vi "EnFlo_Hub.vi"() -> ()   [LabVIEW 2012]
uses:
  Anemometry Sub Vis/Controls/Launch_controls/Open_Calib.ctl
  Anemometry Sub Vis/Controls/Launch_controls/Open_Meas.ctl
  Anemometry Sub Vis/Controls/Launch_controls/Open_Enter_Temp.ctl
  Anemometry Sub Vis/Controls/Launch_controls/Multi_Run_Prog.ctl
  Anemometry Sub Vis/Controls/Launch_controls/EnFlo_arm.ctl
  Anemometry Sub Vis/Controls/Launch_controls/Fast_FID_Valve.ctl
  Anemometry Sub Vis/Controls/Launch_controls/Disp_Setup.ctl
  Anemometry Sub Vis/Controls/Launch_controls/EnFlo_Tun_Setup.ctl
  Anemometry Sub Vis/Controls/Launch_controls/User_Metadata.ctl
  Anemometry Sub Vis/Controls/Launch_controls/Trav_3D_move.ctl
  Anemometry Sub Vis/Controls/Launch_controls/Trav_Space.ctl
  Anemometry Sub Vis/Controls/Launch_controls/Tunnel_speed.ctl
  Anemometry Sub Vis/Controls/Launch_controls/Client_source_control.ctl
  Anemometry Sub Vis/Controls/Launch_controls/Hydrosonic_Manual.ctl
  Anemometry Sub Vis/Controls/Launch_controls/Preference_Panel.ctl
  Anemometry Sub Vis/Controls/Launch_controls/Hot_wire_Calculator.ctl
  Anemometry Sub Vis/Controls/Launch_controls/RW_X_Parker_Config.ctl
  Anemometry Sub Vis/Controls/Launch_controls/LDA_Alignment.ctl
  Anemometry Sub Vis/Controls/Launch_controls/Named_Serial_Comms.ctl
  Anemometry Sub Vis/Controls/Launch_controls/BSA_data_rates.ctl
  Anemometry Sub Vis/Controls/Launch_controls/Serial_Setup.ctl
  Anemometry Sub Vis/Controls/Launch_controls/Post_Process_icon.ctl
  Anemometry Sub Vis/Controls/Launch_controls/Edit_Ascii_file.ctl
  Anemometry Sub Vis/Controls/Launch_controls/Edit_Raw_DF.ctl
  Anemometry Sub Vis/Controls/Launch_controls/Results_file_plotter.ctl
  Anemometry Sub Vis/Controls/Launch_controls/Serial_Port_Names.ctl
  Anemometry Sub Vis/Controls/Launch_controls/Paul.ctl
  Anemometry Sub Vis/Controls/Launch_controls/Tom.ctl
  Anemometry Sub Vis/Controls/Launch_controls/Scani_Valve.ctl
  Anemometry Sub Vis/Controls/Launch_controls/Edit_sever_Channel.ctl
  Anemometry Sub Vis/Controls/Launch_controls/Day_file_plotter.ctl
  Anemometry Sub Vis/Controls/Launch_controls/Plot_Sever_Data.ctl
  Anemometry Sub Vis/Controls/Launch_controls/Adam_Table.ctl
  Anemometry Sub Vis/Controls/Launch_controls/Active_Channel_Control.ctl
  Anemometry Sub Vis/Controls/Setup.ctl
  Anemometry Sub Vis/Controls/Post_Process.ctl
  Anemometry Sub Vis/Controls/Preference_Mode.ctl
  Anemometry Sub Vis/Gen Trav/Trav_mode.ctl
  Anemometry Sub Vis/Controls/User_Specific_mode.ctl
  Anemometry Sub Vis/File/Setup_Filetype.ctl
  Anemometry Sub Vis/Calibration/Calib_mode.ctl
  Anemometry Sub Vis/Controls/Server_Comms.ctl
  Anemometry Sub Vis/Controls/App_Global.ctl
  Anemometry Sub Vis/Globals/Dynamic_call_global.ph.vi
  Anemometry Sub Vis/Globals/Constants_global.vi
  Anemometry Sub Vis/Globals/Preference_global.vi
  Anemometry Sub Vis/Globals/Meas_global.vi
  <vilib>/Platform/browser.llb/Open URL in Default Browser (string).vi
  Anemometry Sub Vis/Globals/Trav_pos_global.vi
  Anemometry Sub Vis/Acquisition/PWA/PWAtasksGLOBAL.vi
  Anemometry Sub Vis/Utilities/Email_transfer_global.vi
panel:
  out "List of ADAM channels to view":string[](array[string])
  out "List of ADAM control channels":string[](array[string])
  out "Analogue Dev Name":string="Dev2"
  out "Numeric":i32
  out "Rig Name":string="EnFlo Tunnel"
  out "All Users":path=path "/System Folder/Preferences/LabVIEW (EnFlo specific)/Meas Setups"
  out "Dummy Measurement":bool
  in  "stop":bool
  in  "Tab Control":T1(tab)
  in  "Tunnel Speed Control":T2
  in  "Traverse Space":T3
  in  "Trav 3D Move":T4 caption="3D Traverse Move"
  in  "User Metadata":T5
  in  "Multi Run Prog":T6
  in  "Enter Temp_Press":T7
  in  "Measurement Prog":T8 caption="Measurement"
  in  "Calibration Prog":T9 caption="Calibration"
  in  "Scani Valve":T10
  in  "LDA Alignment":T11
  in  "Hydrosonic Control":T12
  in  "Fast FID Valve":T13
  in  "Source Control":T14
  in  "Gas Release Setup":T15
  in  "EnFlo Tunnel Setup":T16
  in  "Heater Setup":bool caption="Inlet heater File"
  in  "EnFlo Arm":T17
  in  "EnFlo Tun Display":bool
  in  "Rig_Control":cluster{"Ch Name":string, "Boolean":bool}[](array[cluster])
  in  "ADAM Channels Control":T18 caption="Change Active Channels"
  in  "ADAM Scan Table":T19 caption="Run ADAM Scan Table"
  in  "Edit Server Channel":T20
  in  "Plot Server Channels":T21 caption="Plot Server Data"
  in  "Day Files Plotter":T22 caption="Plot Data From File"
  out "Current Values":cluster{"Ch Name":string, "Numeric":dbl}[](array[cluster])
  in  "Results File Plotter":T23
  in  "Edit Raw Data Files":T24
  in  "Edit ASCII File":T25
  in  "Post Process Raw Data":T26
  in  "Top Level Traverse":bool
  in  "Show Manual Sync":bool
  in  "Sync to server now":bool
  in  "Port Names":T27
  in  "Serial Setup":T28
  in  "LDA Data Rate":T29
  in  "Named Serial Comms":T30
  in  "RW Trav Setup":T31
  in  "Hot Wire Calc":T32
  in  "Preference Panel":T33
  in  "Tom Lawton t.lawton@surrey.ac.uk":T34 caption="For hardware support"
  in  "Paul Hayden p.hayden@surrey.ac.uk":T35 caption="For software support"
  in  "Online Manual":bool
  out "VI Name":string
  out "Iterations":i32
  # "Or give us a call on Tel: 01483 689545"
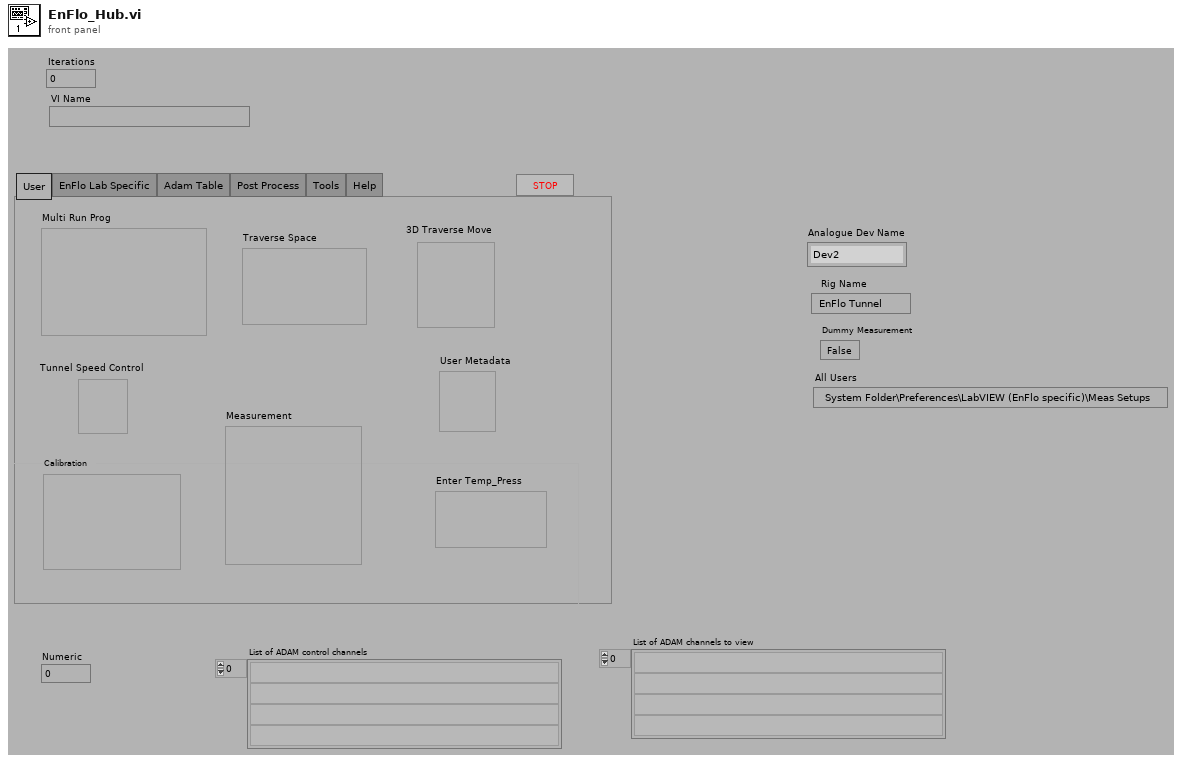
[diagram p1: front panel]
types:
  T1 = enum32{"User", "EnFlo Lab Specific", "Adam Table", "Post Process", "Tools", "Help"}
  T2 = typedef "Tunnel_speed.ctl" = bool
  T3 = typedef "Trav_Space.ctl" = bool
  T4 = typedef "Trav_3D_move.ctl" = bool
  T5 = typedef "User_Metadata.ctl" = bool
  T6 = typedef "Multi_Run_Prog.ctl" = bool
  T7 = typedef "Open_Enter_Temp.ctl" = bool
  T8 = typedef "Open_Meas.ctl" = bool
  T9 = typedef "Open_Calib.ctl" = bool
  T10 = typedef "Scani_Valve.ctl" = bool
  T11 = typedef "LDA_Alignment.ctl" = bool
  T12 = typedef "Hydrosonic_Manual.ctl" = bool
  T13 = typedef "Fast_FID_Valve.ctl" = bool
  T14 = typedef "Client_source_control.ctl" = bool
  T15 = typedef "Disp_Setup.ctl" = bool
  T16 = typedef "EnFlo_Tun_Setup.ctl" = bool
  T17 = typedef "EnFlo_arm.ctl" = bool
  T18 = typedef "Active_Channel_Control.ctl" = bool
  T19 = typedef "Adam_Table.ctl" = bool
  T20 = typedef "Edit_sever_Channel.ctl" = bool
  T21 = typedef "Plot_Sever_Data.ctl" = bool
  T22 = typedef "Day_file_plotter.ctl" = bool
  T23 = typedef "Results_file_plotter.ctl" = bool
  T24 = typedef "Edit_Raw_DF.ctl" = bool
  T25 = typedef "Edit_Ascii_file.ctl" = bool
  T26 = typedef "Post_Process_icon.ctl" = bool
  T27 = typedef "Serial_Port_Names.ctl" = bool
  T28 = typedef "Serial_Setup.ctl" = bool
  T29 = typedef "BSA_data_rates.ctl" = bool
  T30 = typedef "Named_Serial_Comms.ctl" = bool
  T31 = typedef "RW_X_Parker_Config.ctl" = bool
  T32 = typedef "Hot_wire_Calculator.ctl" = bool
  T33 = typedef "Preference_Panel.ctl" = bool
  T34 = typedef "Tom.ctl" = bool
  T35 = typedef "Paul.ctl" = bool
  T36 = typedef "Post_Process.ctl" = enum16{"Take New Data", "Post Process Raw Data File"}
  T37 = typedef "Setup.ctl" = enum16{"Run Program", "Show Setup", "Save Current Setup", "Setup Front Panel"}
  T38 = enum16{"Get Channel Names", "Get Current Value", "Update Channel Value", "Update Channel Description"}
  T39 = enum32{"Invalid", "Standard", "Closed", "Hidden", "Minimized", "Maximized"}
  T40 = typedef "Preference_Mode.ctl" = enum16{"Load Preferences from file", "Save Preferences to file", "Load, Edit then Save"}
  T41 = typedef "User_Specific_mode.ctl" = enum16{"Check VI only", "Run VI"}
  T42 = typedef "Trav_mode.ctl" = enum16{"Move traverse", "Read traverse position", "Teach Position"}
  T43 = typedef "Setup_Filetype.ctl" = enum16{"Measurement Setups", "Calibration Setups", "General", "Results File Plotter Setups", "Speed Calib Tweaks"}
  T44 = enum16{"Load Command File", "Save Command File", "Check Multi Run Prog", "Check Multi Run Prog With Live Moves", "Run Multi Run Prog"}
  T45 = typedef "Calib_mode.ctl" = enum16{"Show Setup", "Take a New Calibration Point", "Refit Curve", "Setup Front Panel"}
  T46 = typedef "Tunnel_Coordinates.ctl" = enum16{"Work in Tunnel Coordinates", "Work in Model Coordinates"}
  T47 = typedef "App_Global.ctl" = enum16{"Read Global", "Write to Global", "Initialise Array"}
  T48 = typedef "App_Ref_Cluster.ctl" = cluster{"Server IP & Port No":string, "Application reference":refnum<vi>}
  T49 = typedef "Server_Comms.ctl" = enum16{"Server Link Healthy", "Do Not Link To Server"}
  T50 = typedef "Ch_description_ADAM.ctl" = cluster{"Ch Name":string, "Type":T51, "Function":T52, "Ch State":T53, "Calibration type":T54, "A":dbl, "B":dbl, "C":dbl, "D":dbl, "Comments":string, "Address":T55, "String":string, "Duty":u16}
  T51 = typedef "Module_type_ADAM.ctl" = string
  T52 = typedef "Function_ADAM.ctl" = enum16{"Analogue Input", "Digital Input", "Event counter", "Event rate", "Analogue Output", "Digital Output", "Relay Output"}
  T53 = typedef "Channel_State.ctl" = enum16{"On", "Off", "Always On", "Always Off"}
  T54 = typedef "Calib_type_ADAM.ctl" = enum16{"Raw", "Bx + A", "Cx^2 + Bx + A", "Dx^3 + Cx^2 + Bx + A", "In Band", "Hi-Tec Q", "Hi-Tec M_dot", "Text"}
  T55 = typedef "Address.ctl" = cluster{"Main":i32, "Ch.":i32, "Sub":i32, "Port Name":string}
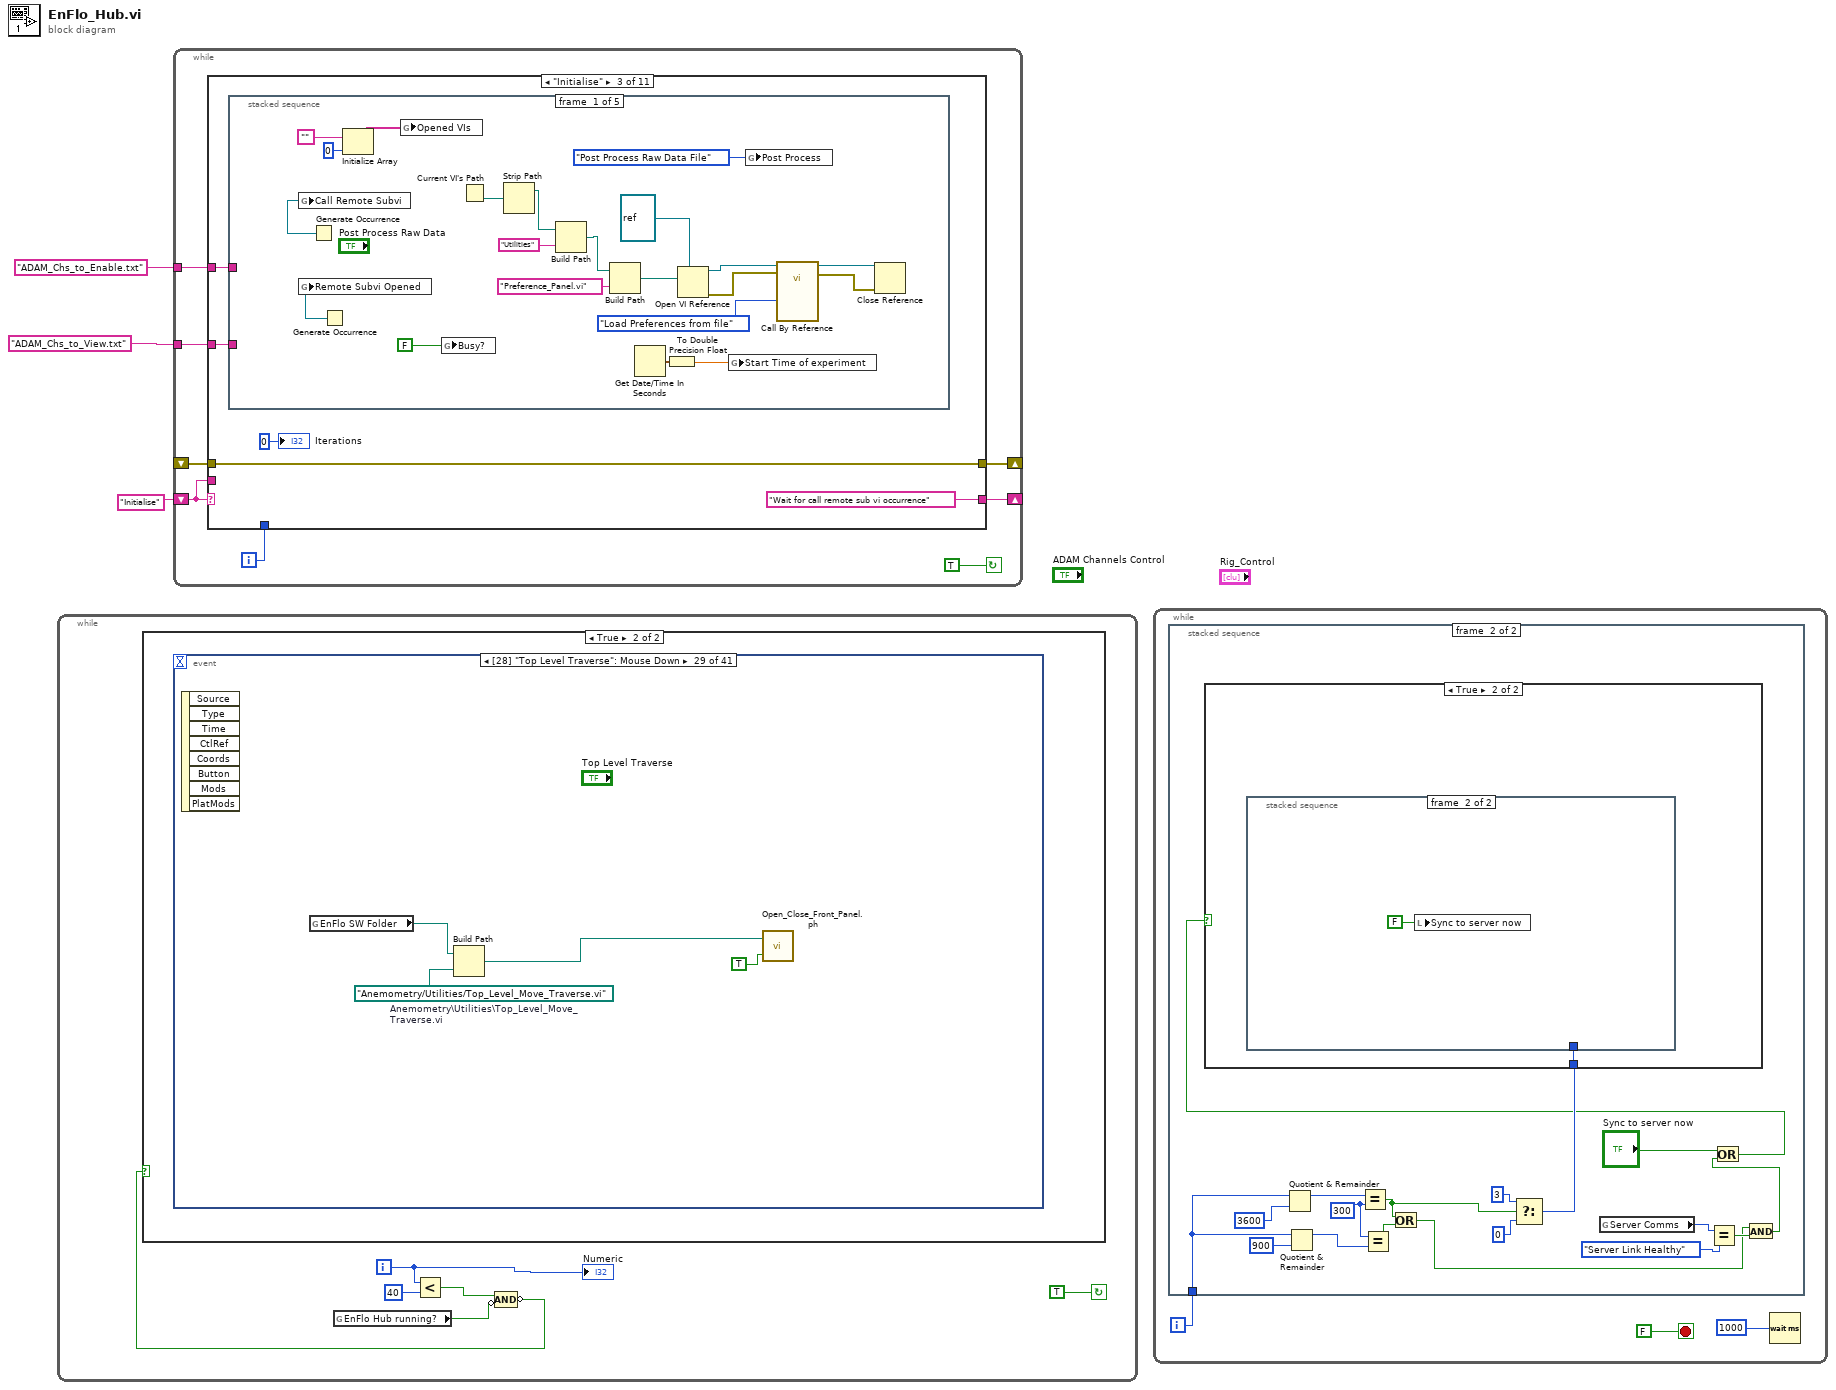
[diagram p0: block diagram]
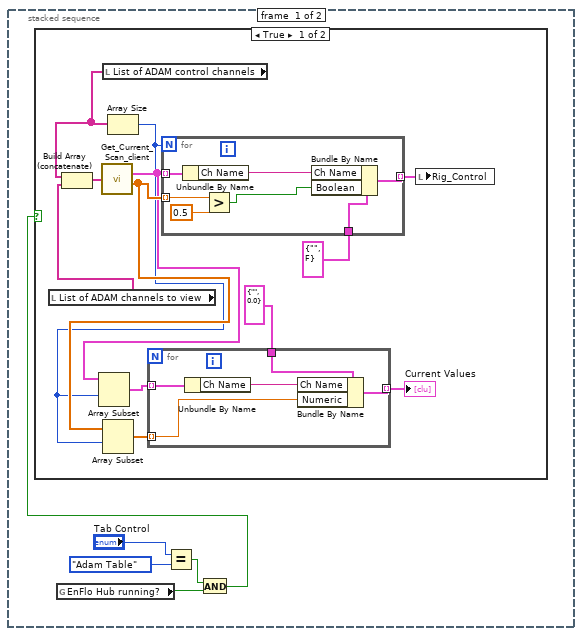
[diagram p2: hidden frame]
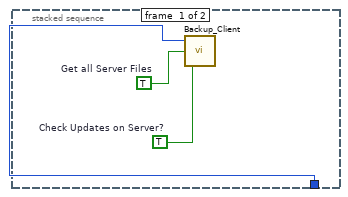
[diagram p5: hidden frame]
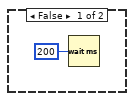
[diagram p6: hidden frame]
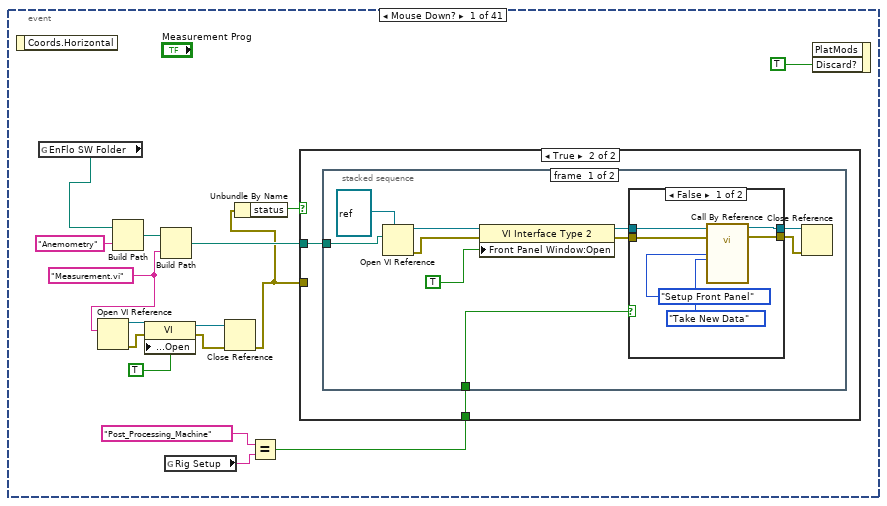
[diagram p7: hidden frame]
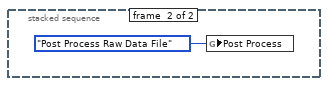
[diagram p10: hidden frame]
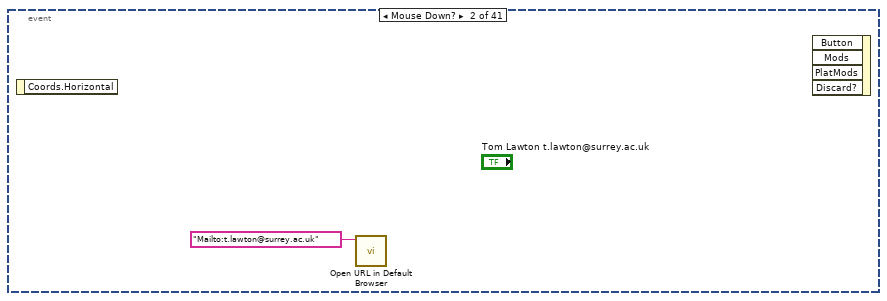
[diagram p11: hidden frame]
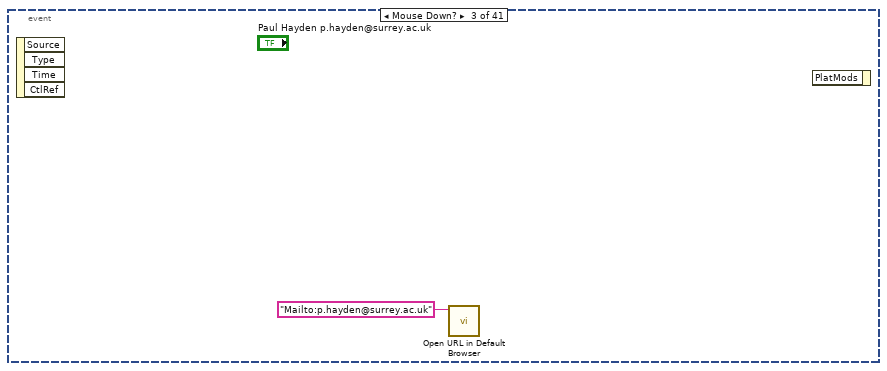
[diagram p12: hidden frame]
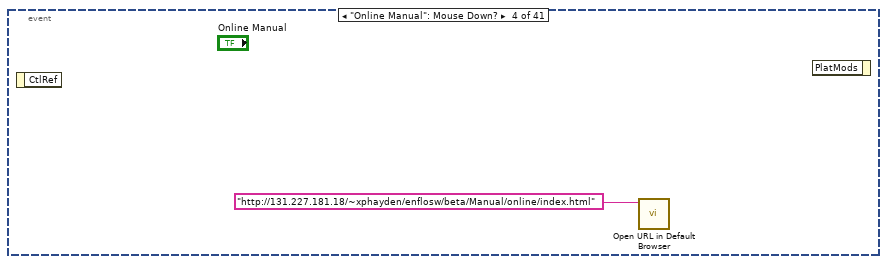
[diagram p13: hidden frame]
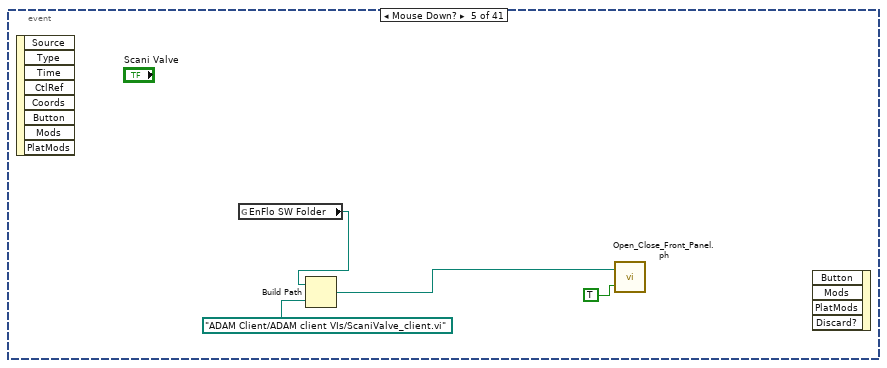
[diagram p14: hidden frame]
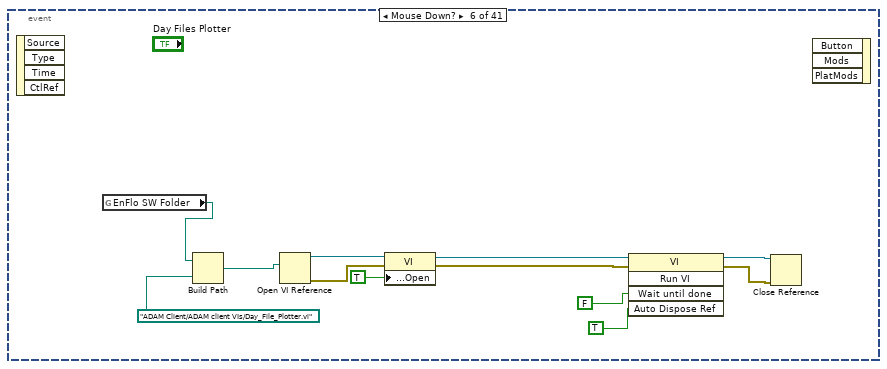
[diagram p15: hidden frame]
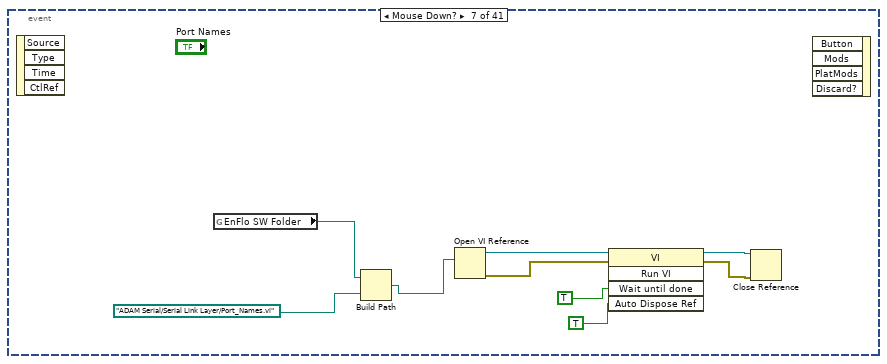
[diagram p16: hidden frame]
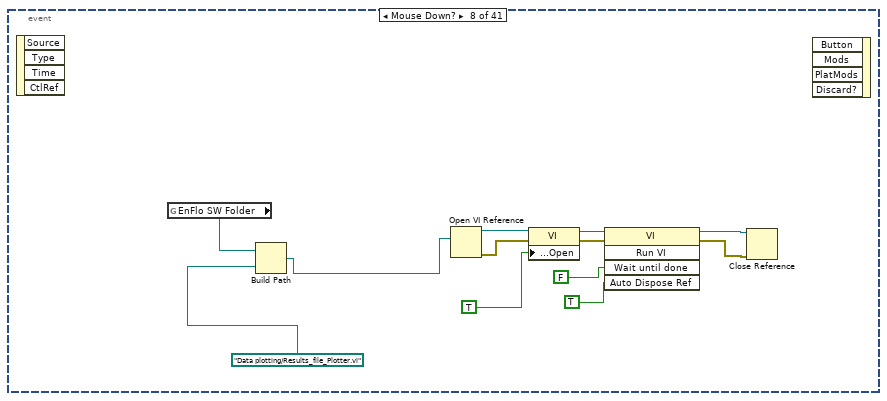
[diagram p17: hidden frame]
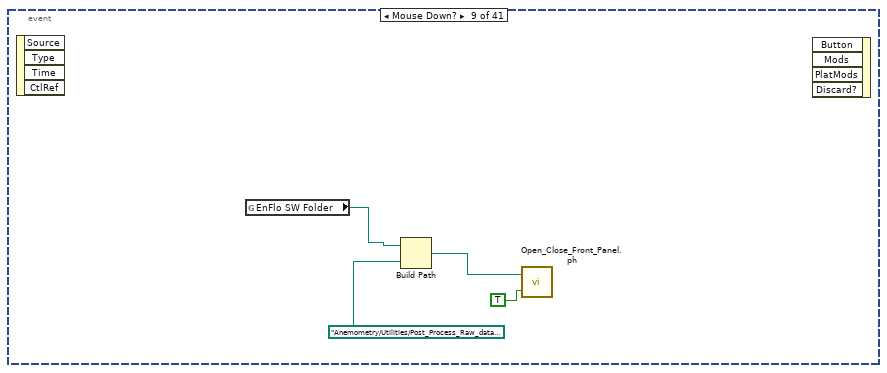
[diagram p18: hidden frame]
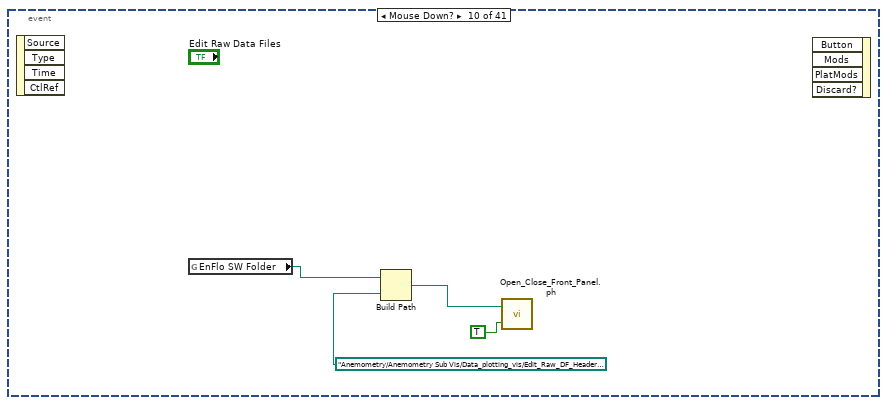
[diagram p19: hidden frame]
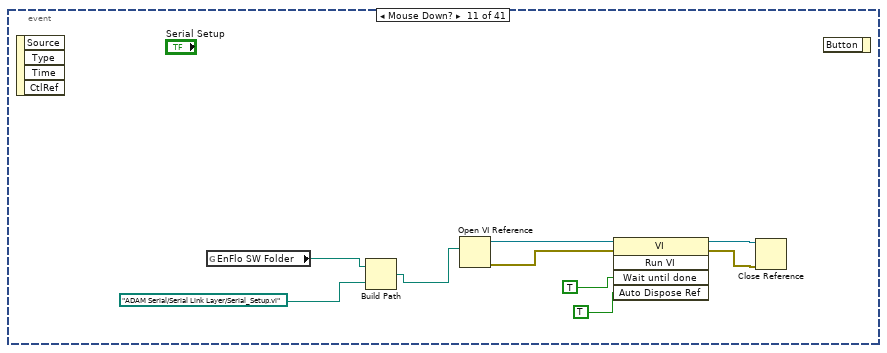
[diagram p20: hidden frame]
diagram:
  n1 = while {
    i -> [w8]
    stop <- TRUE continue-if-true
    n2 = global read "Dynamic_call_global.ph.vi" "EnFlo Hub running?"() -> (w6:bool)
    n3 = Less?(x=w8, y=40) -> (x < y?=w5:bool)
    n4 = Compound Arithmetic op=AND(w5, invert w6) -> (invert w4:bool)
    n5 = case shown="True" w4 {
      frame False {
        n6 = Wait (ms)(milliseconds to wait=u32 200) -> ()  [unwired: 1 out]
      }
      frame True {
        n7 = event shown="[28] \"Top Level Traverse\": Mouse Down" {
          selector: _ -> [_ _ _ _ _ _ _ _ _ _ _ _ _ _ _ _ _ _ _ _ _ _ _ _ _ _ _ _ _ _ _ _ _ _ _ _ _ _ _ _ _]
          dyn-events: _ -> [_ _ _ _ _ _ _ _ _ _ _ _ _ _ _ _ _ _ _ _ _ _ _ _ _ _ _ _ _ _ _ _ _ _ _ _ _ _ _ _ _]
          timeout: _ -> [_ _ _ _ _ _ _ _ _ _ _ _ _ _ _ _ _ _ _ _ _ _ _ _ _ _ _ _ _ _ _ _ _ _ _ _ _ _ _ _ _]
          event Mouse Down? {
            w19 = "Measurement.vi" ("name or relative path")
            n8 = event-data() -> ()  [unwired: 2 out]
            n9 = global read "Constants_global.vi" "EnFlo SW Folder"() -> (w22:path)
            n10 = Open VI Reference(vi path=w19) -> (vi reference=w18:refnum<vi>, error out=w17:errorcluster)  [unwired: 1 in, 4 out]
            n11 = Build Path(base path=w22, name or relative path="Anemometry") -> (appended path=w25:path)
            n12 = property class="VI"(reference=w18, error in=w17, "Front Panel Window:Open"=TRUE) -> (reference out=w15:refnum<vi>, error out=w16:errorcluster)
            n13 = Build Path(base path=w25, name or relative path=w19) -> (appended path=w23:path)
            n14 = global read "Preference_global.vi" "Rig Setup"() -> (w13:string)
            n15 = Close Reference(reference=w15, error in (no error)=w16) -> (error out=w14:errorcluster)
            n16 = Unbundle By Name(w14) -> ("status"=w24:bool)
            n17 = Equal?(x="Post_Processing_Machine" ("Rig Setup"), y=w13) -> (x = y?=w11:bool)
            n18 = case shown="True" w24 {
              tunnel: w23 -> [_ w28]
              tunnel: w14 -> [_ _]
              tunnel: w11 -> [_ w27]
              frame False {
              }
              frame True {
                n19 = stacked-sequence {
                  tunnel: w28 -> [w38 _]
                  tunnel: w27 -> [w29 _]
                  frame #0 {
                    n20 = Open VI Reference(type specifier VI Refnum (for type only)=refnum<vi> refnum, vi path=w38) -> (vi reference=w36:refnum<vi>, error out=w35:errorcluster)  [unwired: 1 in, 3 out]
                    n21 = property class="VI Interface Type 2"(reference=w36, error in=w35, "Front Panel Window:Open"=TRUE) -> (reference out=w31:refnum<vi>, error out=w30:errorcluster)
                    n22 = case shown="False" w29 {
                      tunnel: [w44 w46] -> w34
                      tunnel: [w43 w45] -> w33
                      tunnel: w31 -> [w42 w46]
                      tunnel: w30 -> [w41 w45]
                      frame False {
                        n23 = call-by-ref "?"(reference=w42, error in=w41, "setup"=Setup."Setup Front Panel", "Post Process"=Post_Process."Take New Data") -> (reference out=w44:refnum<vi>, error out=w43:errorcluster)  [unwired: 16 in, 2 out]
                      }
                      frame True {
                      }
                    }
                    n24 = Close Reference(reference=w34, error in (no error)=w33) -> ()  [unwired: 1 out]
                  }
                  frame #1 {
                    n25 = global write "Meas_global.vi" "Post Process"(Post_Process."Post Process Raw Data File" ("Post Process")) -> ()
                  }
                }
              }
            }
            n26 = event-data("Discard?"=TRUE) -> ()  [unwired: 1 in, 2 out]
          }
          event Mouse Down? {
            n27 = event-data() -> ()  [unwired: 2 out]
            n28 = call-poly <vilib>:"Open URL in Default Browser.vi"("URL"="Mailto:t.lawton@surrey.ac.uk") -> ()  [unwired: 1 in, 6 out]
            n29 = event-data() -> ()  [unwired: 1 in, 5 out]
          }
          event Mouse Down? {
            n30 = event-data() -> ()  [unwired: 5 out]
            n31 = call-poly <vilib>:"Open URL in Default Browser.vi"("URL"="Mailto:p.hayden@surrey.ac.uk") -> ()  [unwired: 1 in, 6 out]
            n32 = event-data() -> ()  [unwired: 1 in, 2 out]
          }
          event "Online Manual": Mouse Down? {
            n33 = event-data() -> ()  [unwired: 2 out]
            n34 = call-poly <vilib>:"Open URL in Default Browser.vi"("URL"="http://131.227.181.18/~xphayden/enflosw/beta/Manual/online/index.html") -> ()  [unwired: 1 in, 6 out]
            n35 = event-data() -> ()  [unwired: 1 in, 2 out]
          }
          event Mouse Down? {
            n36 = event-data() -> ()  [unwired: 9 out]
            n37 = global read "Constants_global.vi" "EnFlo SW Folder"() -> (w51:path)
            n38 = Build Path(base path=w51, name or relative path=path "ADAM Client/ADAM client VIs/ScaniValve_client.vi") -> (appended path=w54:path)
            n39 = call "Open_Close_Front_Panel.ph.vi"("Front Panel Window:Open"=TRUE, "VI path"=w54) -> ()  [unwired: 2 out]
            n40 = event-data() -> ()  [unwired: 1 in, 5 out]
          }
          event Mouse Down? {
            n41 = event-data() -> ()  [unwired: 5 out]
            n42 = global read "Constants_global.vi" "EnFlo SW Folder"() -> (w55:path)
            n43 = Build Path(base path=w55, name or relative path=path "ADAM Client/ADAM client VIs/Day_File_Plotter.vi") -> (appended path=w61:path)
            n44 = Open VI Reference(vi path=w61) -> (vi reference=w62:refnum<vi>, error out=w64:errorcluster)  [unwired: 2 in, 3 out]
            n45 = property class="VI"(reference=w62, error in=w64, "Front Panel Window:Open"=TRUE) -> (reference out=w66:refnum<vi>, error out=w65:errorcluster)
            n46 = invoke class="VI" method="Run VI"(reference=w66, error in=w65, "Wait until done"=FALSE, "Auto Dispose Ref"=TRUE) -> (reference out=w57:refnum<vi>, error out=w58:errorcluster)  [unwired: 1 in, 3 out]
            n47 = Close Reference(reference=w57, error in (no error)=w58) -> ()  [unwired: 1 out]
            n48 = event-data() -> ()  [unwired: 1 in, 4 out]
          }
          event Mouse Down? {
            n49 = event-data() -> ()  [unwired: 5 out]
            n50 = global read "Constants_global.vi" "EnFlo SW Folder"() -> (w67:path)
            n51 = Build Path(base path=w67, name or relative path=path "ADAM Serial/Serial Link Layer/Port_Names.vi") -> (appended path=w69:path)
            n52 = Open VI Reference(vi path=w69) -> (vi reference=w74:refnum<vi>, error out=w75:errorcluster)  [unwired: 1 in, 4 out]
            n53 = invoke class="VI" method="Run VI"(reference=w74, error in=w75, "Wait until done"=TRUE, "Auto Dispose Ref"=TRUE) -> (reference out=w70:refnum<vi>, error out=w71:errorcluster)  [unwired: 1 in, 3 out]
            n54 = Close Reference(reference=w70, error in (no error)=w71) -> ()  [unwired: 1 out]
            n55 = event-data() -> ()  [unwired: 1 in, 5 out]
          }
          event Mouse Down? {
            n56 = event-data() -> ()  [unwired: 5 out]
            n57 = global read "Constants_global.vi" "EnFlo SW Folder"() -> (w76:path)
            n58 = Build Path(base path=w76, name or relative path=path "Data plotting/Results_file_Plotter.vi") -> (appended path=w79:path)
            n59 = Open VI Reference(vi path=w79) -> (vi reference=w81:refnum<vi>, error out=w78:errorcluster)  [unwired: 1 in, 4 out]
            n60 = property class="VI"(reference=w81, error in=w78, "Front Panel Window:Open"=TRUE) -> (reference out=w82:refnum<vi>, error out=w83:errorcluster)
            n61 = invoke class="VI" method="Run VI"(reference=w82, error in=w83, "Wait until done"=FALSE, "Auto Dispose Ref"=TRUE) -> (reference out=w84:refnum<vi>, error out=w85:errorcluster)  [unwired: 1 in, 3 out]
            n62 = Close Reference(reference=w84, error in (no error)=w85) -> ()  [unwired: 1 out]
            n63 = event-data() -> ()  [unwired: 1 in, 5 out]
          }
          event Mouse Down? {
            n64 = event-data() -> ()  [unwired: 5 out]
            n65 = global read "Constants_global.vi" "EnFlo SW Folder"() -> (w88:path)
            n66 = Build Path(base path=w88, name or relative path=path "Anemometry/Utilities/Post_Process_Raw_data.vi") -> (appended path=w90:path)
            n67 = call "Open_Close_Front_Panel.ph.vi"("Front Panel Window:Open"=TRUE, "VI path"=w90) -> ()  [unwired: 2 out]
            n68 = event-data() -> ()  [unwired: 1 in, 5 out]
          }
          event Mouse Down? {
            n69 = event-data() -> ()  [unwired: 5 out]
            n70 = global read "Constants_global.vi" "EnFlo SW Folder"() -> (w92:path)
            n71 = Build Path(base path=w92, name or relative path=path "Anemometry/Anemometry Sub Vis/Data_plotting_vis/Edit_Raw_DF_Header.vi") -> (appended path=w94:path)
            n72 = call "Open_Close_Front_Panel.ph.vi"("Front Panel Window:Open"=TRUE, "VI path"=w94) -> ()  [unwired: 2 out]
            n73 = event-data() -> ()  [unwired: 1 in, 5 out]
          }
          event Mouse Down? {
            n74 = event-data() -> ()  [unwired: 5 out]
            n75 = global read "Constants_global.vi" "EnFlo SW Folder"() -> (w96:path)
            n76 = Build Path(base path=w96, name or relative path=path "ADAM Serial/Serial Link Layer/Serial_Setup.vi") -> (appended path=w98:path)
            n77 = Open VI Reference(vi path=w98) -> (vi reference=w103:refnum<vi>, error out=w104:errorcluster)  [unwired: 1 in, 4 out]
            n78 = invoke class="VI" method="Run VI"(reference=w103, error in=w104, "Wait until done"=TRUE, "Auto Dispose Ref"=TRUE) -> (reference out=w99:refnum<vi>, error out=w100:errorcluster)  [unwired: 1 in, 3 out]
            n79 = Close Reference(reference=w99, error in (no error)=w100) -> ()  [unwired: 1 out]
            n80 = event-data() -> ()  [unwired: 1 in, 2 out]
          }
          event Mouse Down? {
            n81 = event-data() -> ()  [unwired: 5 out]
            n82 = global read "Constants_global.vi" "EnFlo SW Folder"() -> (w106:path)
            n83 = Build Path(base path=w106, name or relative path=path "ADAM Serial/Serial Link Layer/Named_Serial_Comms.vi") -> (appended path=w108:path)
            n84 = call "Open_Close_Front_Panel.ph.vi"("Front Panel Window:Open"=TRUE, "VI path"=w108) -> ()  [unwired: 2 out]
            n85 = event-data() -> ()  [unwired: 1 in, 5 out]
          }
          event Mouse Down? {
            n86 = event-data() -> ()  [unwired: 5 out]
            n87 = global read "Constants_global.vi" "EnFlo SW Folder"() -> (w109:path)
            n88 = Build Path(base path=w109, name or relative path=path "Anemometry/Anemometry Sub Vis/LDA/LDA_data_rate.vi") -> (appended path=w111:path)
            n89 = call "Open_Close_Front_Panel.ph.vi"("Front Panel Window:Open"=TRUE, "VI path"=w111) -> ()  [unwired: 2 out]
            n90 = event-data() -> ()  [unwired: 1 in, 2 out]
          }
          event Mouse Down? {
            n91 = event-data() -> ()  [unwired: 5 out]
            n92 = global read "Constants_global.vi" "EnFlo SW Folder"() -> (w123:path)
            n93 = Build Path(base path=w123, name or relative path=path "ADAM Client/ADAM client VIs/Control_Channel_Status.vi") -> (appended path=w113:path)
            n94 = Open VI Reference(vi path=w113) -> (vi reference=w116:refnum<vi>, error out=w114:errorcluster)  [unwired: 1 in, 4 out]
            n95 = property class="VI"(reference=w116, error in=w114, "Front Panel Window:Open"=TRUE) -> (reference out=w117:refnum<vi>, error out=w118:errorcluster)
            n96 = invoke class="VI" method="Run VI"(reference=w117, error in=w118, "Wait until done"=FALSE, "Auto Dispose Ref"=TRUE) -> (reference out=w119:refnum<vi>, error out=w120:errorcluster)  [unwired: 1 in, 3 out]
            n97 = Close Reference(reference=w119, error in (no error)=w120) -> ()  [unwired: 1 out]
            n98 = event-data() -> ()  [unwired: 1 in, 2 out]
          }
          event Mouse Down? {
            n99 = event-data() -> ()  [unwired: 5 out]
            n100 = global read "Constants_global.vi" "EnFlo SW Folder"() -> (w125:path)
            n101 = Build Path(base path=w125, name or relative path=path "Anemometry/Utilities/LDA_Beam_Alignment.vi") -> (appended path=w127:path)
            n102 = call "Open_Close_Front_Panel.ph.vi"("Front Panel Window:Open"=TRUE, "VI path"=w127) -> ()  [unwired: 2 out]
            n103 = event-data() -> ()  [unwired: 1 in, 5 out]
          }
          event Mouse Down? {
            w130 = FALSE  # Wait until done
            n104 = event-data() -> ()  [unwired: 5 out]
            n105 = call "Run_Enter_Temp.vi"("Wait until done"=w130) -> ()  [unwired: 1 out]
            n106 = event-data("Discard?"=TRUE) -> ()  [unwired: 1 in, 4 out]
          }
          event Mouse Down? {
            n107 = event-data() -> ()  [unwired: 5 out]
            n108 = global read "Constants_global.vi" "EnFlo SW Folder"() -> (w131:path)
            n109 = Build Path(base path=w131, name or relative path=path "Anemometry/Utilities/Edit_ASCI_file.vi") -> (appended path=w134:path)
            n110 = call "Open_Close_Front_Panel.ph.vi"("Front Panel Window:Open"=TRUE, "VI path"=w134) -> ()  [unwired: 2 out]
            n111 = event-data() -> ()  [unwired: 1 in, 5 out]
          }
          event "Heater Setup": Mouse Down? {
            n112 = event-data() -> ()  [unwired: 5 out]
            n113 = global read "Constants_global.vi" "EnFlo SW Folder"() -> (w135:path)
            n114 = Build Path(base path=w135, name or relative path=path "Anemometry/Utilities/Create_Heater_Setpoints_File.vi") -> (appended path=w138:path)
            n115 = call "Open_Close_Front_Panel.ph.vi"("Front Panel Window:Open"=TRUE, "VI path"=w138) -> ()  [unwired: 2 out]
            n116 = event-data() -> ()  [unwired: 1 in, 5 out]
          }
          event Mouse Down? {
            n117 = event-data() -> ()  [unwired: 5 out]
            n118 = global read "Constants_global.vi" "EnFlo SW Folder"() -> (w139:path)
            n119 = Build Path(base path=w139, name or relative path=path "ADAM Client/Sub VIs/Gas_Release_Control.vi") -> (appended path=w142:path)
            n120 = call "Open_Close_Front_Panel.ph.vi"("Front Panel Window:Open"=TRUE, "VI path"=w142) -> ()  [unwired: 2 out]
            n121 = event-data() -> ()  [unwired: 1 in, 5 out]
          }
          event Mouse Down? {
            n122 = event-data() -> ()  [unwired: 5 out]
            n123 = global read "Constants_global.vi" "EnFlo SW Folder"() -> (w143:path)
            n124 = Build Path(base path=w143, name or relative path=path "ADAM Client/ADAM client VIs/Edit_Server_Channel.vi") -> (appended path=w153:path)
            n125 = Open VI Reference(type specifier VI Refnum (for type only)=refnum<vi> refnum, vi path=w153) -> (vi reference=w146:refnum<vi>, error out=w147:errorcluster)  [unwired: 1 in, 3 out]
            n126 = property class="VI Interface Type 3"(reference=w146, error in=w147, "Front Panel Window:Open"=TRUE) -> (reference out=w149:refnum<vi>, error out=w150:errorcluster)
            n127 = call-by-ref "?"(reference=w149, error in=w150, "Mode"=T38."Get Channel Names") -> (reference out=w151:refnum<vi>, error out=w152:errorcluster)  [unwired: 5 in]
            n128 = Close Reference(reference=w151, error in (no error)=w152) -> ()  [unwired: 1 out]
            n129 = event-data() -> ()  [unwired: 1 in, 5 out]
          }
          event "EnFlo Tun Display": Mouse Down? {
            n130 = event-data() -> ()  [unwired: 9 out]
            n131 = global read "Constants_global.vi" "EnFlo SW Folder"() -> (w166:path)
            n132 = Build Path(base path=w166, name or relative path=path "Anemometry/Utilities/EnFlo_Tunnel_Display.vi") -> (appended path=w161:path)
            n133 = Open VI Reference(vi path=w161) -> (vi reference=w160:refnum<vi>, error out=w159:errorcluster)  [unwired: 5 in]
            n134 = invoke class="VI" method="FP.Open"(reference=w160, error in=w159, "Activate"=TRUE ("Activate?"), "State"=T39."Standard") -> (reference out=w158:refnum<vi>, error out=w157:errorcluster)  [unwired: 1 in, 3 out]
            n135 = invoke class="VI" method="Run VI"(reference=w158, error in=w157, "Wait until done"=FALSE ("Wait Until Done"), "Auto Dispose Ref"=FALSE ("Wait until done")) -> (reference out=w162:refnum<vi>, error out=w163:errorcluster)  [unwired: 1 in, 3 out]
            n136 = Close Reference(reference=w162, error in (no error)=w163) -> ()  [unwired: 1 out]
            n137 = event-data() -> ()  [unwired: 5 in, 1 out]
          }
          event Mouse Down? {
            n138 = event-data() -> ()  [unwired: 5 out]
            n139 = global read "Constants_global.vi" "EnFlo SW Folder"() -> (w168:path)
            n140 = Build Path(base path=w168, name or relative path=path "ADAM Client/ADAM client VIs/Set_Tunnel_Speed.vi") -> (appended path=w171:path)
            n141 = call "Open_Close_Front_Panel.ph.vi"("Front Panel Window:Open"=TRUE, "VI path"=w171) -> ()  [unwired: 2 out]
            n142 = event-data() -> ()  [unwired: 1 in, 5 out]
          }
          event Mouse Down? {
            n143 = event-data() -> ()  [unwired: 5 out]
            n144 = global read "Constants_global.vi" "EnFlo SW Folder"() -> (w172:path)
            n145 = Build Path(base path=w172, name or relative path=path "ADAM Client/ADAM client VIs/Plot_Server_Data.vi") -> (appended path=w175:path)
            n146 = Open VI Reference(vi path=w175) -> (vi reference=w177:refnum<vi>, error out=w174:errorcluster)  [unwired: 1 in, 4 out]
            n147 = property class="VI"(reference=w177, error in=w174, "Front Panel Window:Open"=TRUE) -> (reference out=w178:refnum<vi>, error out=w179:errorcluster)
            n148 = invoke class="VI" method="Run VI"(reference=w178, error in=w179, "Wait until done"=FALSE, "Auto Dispose Ref"=TRUE) -> (reference out=w180:refnum<vi>, error out=w181:errorcluster)  [unwired: 1 in, 3 out]
            n149 = Close Reference(reference=w180, error in (no error)=w181) -> ()  [unwired: 1 out]
            n150 = event-data() -> ()  [unwired: 1 in, 5 out]
          }
          event Mouse Down? {
            n151 = event-data() -> ()  [unwired: 5 out]
            n152 = Two Button Dialog(message="Are you sure that you want to Run the ADAM Scan table on this machine?", 1:"Run" ("F button name (\"Cancel\")"), 2:"Cancel" ("T button name (\"OK\")")) -> (T button?=w185:bool)
            n153 = case shown="False" w185 {
              frame False {
                n154 = global read "Constants_global.vi" "EnFlo SW Folder"() -> (w188:path)
                n155 = Build Path(base path=w188, name or relative path=path "ADAM Server/ADAM_scan_table.vi") -> (appended path=w191:path)
                n156 = Open VI Reference(vi path=w191) -> (vi reference=w193:refnum<vi>, error out=w190:errorcluster)  [unwired: 1 in, 4 out]
                n157 = property class="VI"(reference=w193, error in=w190, "Front Panel Window:Open"=TRUE) -> (reference out=w194:refnum<vi>, error out=w195:errorcluster)
                n158 = invoke class="VI" method="Run VI"(reference=w194, error in=w195, "Wait until done"=FALSE, "Auto Dispose Ref"=TRUE) -> (reference out=w196:refnum<vi>, error out=w197:errorcluster)  [unwired: 1 in, 3 out]
                n159 = Close Reference(reference=w196, error in (no error)=w197) -> ()  [unwired: 1 out]
              }
              frame True {
              }
            }
            n160 = event-data() -> ()  [unwired: 1 in, 2 out]
          }
          event Mouse Down? {
            n161 = event-data() -> ()  [unwired: 5 out]
            n162 = global read "Constants_global.vi" "EnFlo SW Folder"() -> (w202:path)
            n163 = Build Path(base path=w202, name or relative path=path "ADAM Serial/Instrument drivers/Traverses/~subVIs/Read_Write_Trav_Config.vi") -> (appended path=w203:path)
            n164 = Build Path(base path=w202, name or relative path=path "ADAM Serial/Instrument drivers/Traverses/~subVIs/DriveConfigGlobal.vi") -> (appended path=w204:path)
            n165 = flat-sequence {
              tunnel: w204 -> [w205]
              tunnel: w203 -> [w207]
              frame #0 {
                n166 = call "Open_Close_Front_Panel.ph.vi"("Front Panel Window:Open"=TRUE, "VI path"=w205) -> ()  [unwired: 2 out]
              }
              frame #1 {
                n167 = call "Open_Close_Front_Panel.ph.vi"("Front Panel Window:Open"=TRUE, "VI path"=w207) -> ()  [unwired: 2 out]
              }
            }
            n168 = event-data() -> ()  [unwired: 1 in, 5 out]
          }
          event Mouse Down? {
            n169 = event-data() -> ()  [unwired: 5 out]
            n170 = global read "Constants_global.vi" "EnFlo SW Folder"() -> (w209:path)
            n171 = Build Path(base path=w209, name or relative path=path "Anemometry/Utilities/Hot_wire_Calculator.vi") -> (appended path=w212:path)
            n172 = call "Open_Close_Front_Panel.ph.vi"("Front Panel Window:Open"=TRUE, "VI path"=w212) -> ()  [unwired: 2 out]
            n173 = event-data() -> ()  [unwired: 1 in, 5 out]
          }
          event "Show Manual Sync": Mouse Down {
            w215 = path "Anemometry/Utilities/EnFlo_Data_Sync_Manual.vi"  # Anemometry\Utilities\EnFlo_Data_Sync_Manual.vi
            n174 = event-data() -> ()  [unwired: 9 out]
            n175 = global read "Constants_global.vi" "EnFlo SW Folder"() -> (w213:path)
            n176 = Build Path(base path=w213, name or relative path=w215) -> (appended path=w216:path)
            n177 = call "Open_Close_Front_Panel.ph.vi"("Front Panel Window:Open"=TRUE, "VI path"=w216) -> ()  [unwired: 2 out]
          }
          event Mouse Down? {
            n178 = event-data() -> ()  [unwired: 5 out]
            n179 = global read "Constants_global.vi" "EnFlo SW Folder"() -> (w217:path)
            n180 = Build Path(base path=w217, name or relative path=path "Anemometry/Utilities/Hydrosonic_Manual.vi") -> (appended path=w220:path)
            n181 = call "Open_Close_Front_Panel.ph.vi"("Front Panel Window:Open"=TRUE, "VI path"=w220) -> ()  [unwired: 2 out]
            n182 = event-data() -> ()  [unwired: 1 in, 5 out]
          }
          event "Top Level Traverse": Mouse Down {
            w223 = path "Anemometry/Utilities/Top_Level_Move_Traverse.vi"  # Anemometry\Utilities\Top_Level_Move_Traverse.vi
            n183 = event-data() -> ()  [unwired: 9 out]
            n184 = global read "Constants_global.vi" "EnFlo SW Folder"() -> (w221:path)
            n185 = Build Path(base path=w221, name or relative path=w223) -> (appended path=w224:path)
            n186 = call "Open_Close_Front_Panel.ph.vi"("Front Panel Window:Open"=TRUE, "VI path"=w224) -> ()  [unwired: 2 out]
          }
          event Mouse Down? {
            n187 = event-data() -> ()  [unwired: 5 out]
            n188 = global read "Constants_global.vi" "EnFlo SW Folder"() -> (w225:path)
            n189 = Build Path(base path=w225, name or relative path=path "ADAM Client/ADAM client VIs/Fast_FID_Valve_Control.vi") -> (appended path=w228:path)
            n190 = call "Open_Close_Front_Panel.ph.vi"("Front Panel Window:Open"=TRUE, "VI path"=w228) -> ()  [unwired: 2 out]
            n191 = event-data() -> ()  [unwired: 1 in, 5 out]
          }
          event Mouse Down? {
            n192 = event-data() -> ()  [unwired: 5 out]
            n193 = global read "Constants_global.vi" "EnFlo SW Folder"() -> (w229:path)
            n194 = Build Path(base path=w229, name or relative path=path "Anemometry/Utilities/Preference_Panel.vi") -> (appended path=w238:path)
            n195 = Open VI Reference(type specifier VI Refnum (for type only)=refnum<vi> refnum, vi path=w238) -> (vi reference=w231:refnum<vi>, error out=w232:errorcluster)  [unwired: 1 in, 3 out]
            n196 = property class="VI Interface Type 4"(reference=w231, error in=w232, "Front Panel Window:Open"=TRUE) -> (reference out=w234:refnum<vi>, error out=w235:errorcluster)
            n197 = call-by-ref "?"(reference=w234, error in=w235, "Mode"=Preference_Mode."Load, Edit then Save") -> (reference out=w236:refnum<vi>, error out=w237:errorcluster)
            n198 = Close Reference(reference=w236, error in (no error)=w237) -> ()  [unwired: 1 out]
            n199 = event-data("Discard?"=TRUE) -> ()  [unwired: 1 in, 4 out]
          }
          event Mouse Down? {
            n200 = event-data() -> ()  [unwired: 5 out]
            n201 = global read "Constants_global.vi" "EnFlo SW Folder"() -> (w245:path)
            n202 = Build Path(base path=w245, name or relative path=path "ADAM Client/Sub VIs/Gas_Setup.vi") -> (appended path=w252:path)
            n203 = Open VI Reference(type specifier VI Refnum (for type only)=refnum<vi> refnum, vi path=w252) -> (vi reference=w248:refnum<vi>, error out=w249:errorcluster)  [unwired: 1 in, 3 out]
            n204 = property class="VI Interface Type 5"(reference=w248, error in=w249, "Front Panel Window:Open"=TRUE) -> (reference out=w253:refnum<vi>, error out=w251:errorcluster)
            n205 = call-by-ref "?"(reference=w253, error in=w251) -> (reference out=w243:refnum<vi>, error out=w242:errorcluster)  [unwired: 9 in]
            n206 = Close Reference(reference=w243, error in (no error)=w242) -> ()  [unwired: 1 out]
            n207 = event-data("Discard?"=TRUE) -> ()  [unwired: 1 in, 4 out]
          }
          event Mouse Down? {
            n208 = event-data() -> ()  [unwired: 5 out]
            n209 = global read "Constants_global.vi" "EnFlo SW Folder"() -> (w257:path)
            n210 = Build Path(base path=w257, name or relative path=path "ADAM Client/Sub VIs/User_Metadata.vi") -> (appended path=w264:path)
            n211 = Open VI Reference(type specifier VI Refnum (for type only)=refnum<vi> refnum, vi path=w264) -> (vi reference=w260:refnum<vi>, error out=w261:errorcluster)  [unwired: 1 in, 3 out]
            n212 = property class="VI Interface Type 5"(reference=w260, error in=w261, "Front Panel Window:Open"=TRUE) -> (reference out=w265:refnum<vi>, error out=w263:errorcluster)
            n213 = call-by-ref "?"(reference=w265, error in=w263) -> (reference out=w255:refnum<vi>, error out=w254:errorcluster)  [unwired: 9 in]
            n214 = Close Reference(reference=w255, error in (no error)=w254) -> ()  [unwired: 1 out]
            n215 = event-data("Discard?"=TRUE) -> ()  [unwired: 1 in, 4 out]
          }
          event Mouse Down? {
            n216 = event-data() -> ()  [unwired: 5 out]
            n217 = global read "Constants_global.vi" "EnFlo SW Folder"() -> (w271:path)
            n218 = Build Path(base path=w271, name or relative path=path "ADAM Client/Sub VIs/EnFlo_Tunnel_Setup.vi") -> (appended path=w274:path)
            n219 = Open VI Reference(type specifier VI Refnum (for type only)=refnum<vi> refnum, vi path=w274) -> (vi reference=w268:refnum<vi>, error out=w267:errorcluster)  [unwired: 1 in, 3 out]
            n220 = call-by-ref "?"(reference=w268, error in=w267) -> (reference out=w270:refnum<vi>, error out=w269:errorcluster)  [unwired: 9 in]
            n221 = Close Reference(reference=w270, error in (no error)=w269) -> ()  [unwired: 1 out]
            n222 = event-data("Discard?"=TRUE) -> ()  [unwired: 1 in, 4 out]
          }
          event Mouse Down? {
            w285 = TRUE  # Show Panel?
            n223 = event-data() -> ()  [unwired: 5 out]
            n224 = global read "Constants_global.vi" "EnFlo SW Folder"() -> (w280:path)
            n225 = Build Path(base path=w280, name or relative path=path "Anemometry/Anemometry Sub Vis/Gen Trav/Traverse_Space.vi") -> (appended path=w283:path)
            n226 = global read "Trav_pos_global.vi" "Default Traverse Setup"() -> (w275:string)
            n227 = Open VI Reference(type specifier VI Refnum (for type only)=refnum<vi> refnum, vi path=w283) -> (vi reference=w284:refnum<vi>, error out=w276:errorcluster)  [unwired: 1 in, 3 out]
            n228 = call-by-ref "?"(reference=w284, error in=w276, "Show Panel?"=w285, "Traverse Setup"=w275) -> (reference out=w278:refnum<vi>, error out=w277:errorcluster)  [unwired: 8 in, 1 out]
            n229 = Close Reference(reference=w278, error in (no error)=w277) -> ()  [unwired: 1 out]
            n230 = event-data("Discard?"=TRUE) -> ()  [unwired: 1 in, 4 out]
          }
          event Mouse Down? {
            n231 = event-data() -> ()  [unwired: 5 out]
            n232 = global read "Constants_global.vi" "EnFlo SW Folder"() -> (w287:path)
            n233 = Build Path(base path=w287, name or relative path=path "Anemometry/Anemometry Sub Vis/Traverse vi's/EnFlo Tunnel specific/Check_EnFlo_Arm.vi") -> (appended path=w289:path)
            n234 = call "Open_Close_Front_Panel.ph.vi"("Front Panel Window:Open"=TRUE, "VI path"=w289) -> ()  [unwired: 2 out]
            n235 = event-data() -> ()  [unwired: 1 in, 2 out]
          }
          event Mouse Down? {
            n236 = event-data() -> ()  [unwired: 5 out]
            n237 = global read "Constants_global.vi" "EnFlo SW Folder"() -> (w297:path)
            n238 = Build Path(base path=w297, name or relative path=path "Anemometry/Anemometry Sub Vis/Gen Trav/3D_Traverse_move.vi") -> (appended path=w294:path)
            n239 = Strip Path(path=w294) -> (name=w293:string)  [unwired: 1 out]
            n240 = Open VI Reference(vi path=w293) -> (vi reference=w295:refnum<vi>, error out=w296:errorcluster)  [unwired: 1 in, 4 out]
            n241 = property class="VI"(reference=w295, error in=w296) -> (reference out=w291:refnum<vi>, error out=w290:errorcluster, "Front Panel Window:Open"=w292:bool)
            n242 = case shown="False" w292 {
              tunnel: w294 -> [w299 _]
              tunnel: w291 -> [_ w316]
              tunnel: w290 -> [_ w315]
              frame False {
                n243 = global read "Trav_pos_global.vi" "Work in Tunnel Coordinates?"() -> (w309:T46)
                n244 = global read "Trav_pos_global.vi" "Default Traverse Setup"() -> (w307:string)
                n245 = Open VI Reference(type specifier VI Refnum (for type only)=refnum<vi> refnum, vi path=w299) -> (vi reference=w303:refnum<vi>, error out=w304:errorcluster)  [unwired: 1 in, 3 out]
                n246 = property class="VI Interface Type 6"(reference=w303, error in=w304, "Front Panel Window:Open"=TRUE) -> (reference out=w300:refnum<vi>, error out=w301:errorcluster)
                n247 = call-by-ref "?"(reference=w300, error in=w301, "Mode"=Trav_mode."Read traverse position", "Work in Tunnel Coordinates"=w309, "Simulate/Run"=User_Specific_mode."Run VI", "Traverse name"=w307) -> (reference out=w305:refnum<vi>, error out=w306:errorcluster)  [unwired: 9 in, 3 out]
                n248 = Close Reference(reference=w305, error in (no error)=w306) -> ()  [unwired: 1 out]
              }
              frame True {
                n249 = property class="VI"(reference=w316, error in=w315, "Front Panel Window:Open"=TRUE) -> (reference out=w314:refnum<vi>, error out=w313:errorcluster)
                n250 = Close Reference(reference=w314, error in (no error)=w313) -> ()  [unwired: 1 out]
              }
            }
            n251 = event-data() -> ()  [unwired: 1 in, 5 out]
          }
          event Mouse Down? {
            n252 = event-data() -> ()  [unwired: 5 out]
            n253 = Open VI Reference(vi path="Multi_Run_Prog.vi") -> (vi reference=w322:refnum<vi>, error out=w321:errorcluster)  [unwired: 1 in, 4 out]
            n254 = property class="VI"(reference=w322, error in=w321, "Front Panel Window:Open"=TRUE) -> (reference out=w319:refnum<vi>, error out=w320:errorcluster)
            n255 = Close Reference(reference=w319, error in (no error)=w320) -> (error out=w317:errorcluster)
            n256 = Unbundle By Name(w317) -> ("status"=w324:bool)
            n257 = case shown="True" w324 {
              frame False {
              }
              frame True {
                n258 = global read "Constants_global.vi" "EnFlo SW Folder"() -> (w332:path)
                n259 = call "Setup_Filepath.vi"("Setup File Type"=Setup_Filetype."General", "Filename in"="Multi_Run_Filename.txt" ("name or relative path")) -> ("Filename Out"=w325:path)  [unwired: 1 out]
                n260 = Build Path(base path=w332, name or relative path=path "Anemometry/Multi_Run_Prog.vi") -> (appended path=w331:path)
                n261 = call "Read_File_Simple.vi"("Filename"=w325) -> ("string"=w330:string)  [unwired: 2 in, 7 out]
                n262 = String To Path(string=w330) -> (path=w328:path)
                n263 = call "Does_file_exist_(simple).vi"("Pathname"=w328) -> ("exists?"=w329:bool)
                n264 = case shown="False" w329 {
                  tunnel: w331 -> [w334 w346]
                  tunnel: w328 -> [_ w343]
                  frame False {
                    n265 = call "Open_Close_Front_Panel.ph.vi"("Front Panel Window:Open"=TRUE, "VI path"=w334) -> ()  [unwired: 2 out]
                  }
                  frame True {
                    n266 = Open VI Reference(type specifier VI Refnum (for type only)=refnum<vi> refnum, vi path=w346) -> (vi reference=w342:refnum<vi>, error out=w341:errorcluster)  [unwired: 1 in, 3 out]
                    n267 = property class="VI Interface Type 7"(reference=w342, error in=w341, "Front Panel Window:Open"=TRUE) -> (reference out=w339:refnum<vi>, error out=w340:errorcluster)
                    n268 = call-by-ref "?"(reference=w339, error in=w340, "Command filename"=w343, "Setup mode"=T44."Load Command File") -> (reference out=w338:refnum<vi>, error out=w337:errorcluster)  [unwired: 18 in]
                    n269 = Close Reference(reference=w338, error in (no error)=w337) -> ()  [unwired: 1 out]
                  }
                }
              }
            }
            n270 = event-data() -> ()  [unwired: 1 in, 5 out]
          }
          event Mouse Down? {
            w348 = "Calibration.vi" ("name or relative path")
            n271 = event-data() -> ()  [unwired: 5 out]
            n272 = global read "Constants_global.vi" "EnFlo SW Folder"() -> (w354:path)
            n273 = Open VI Reference(vi path=w348) -> (vi reference=w352:refnum<vi>, error out=w351:errorcluster)  [unwired: 1 in, 4 out]
            n274 = Build Path(base path=w354, name or relative path="Anemometry") -> (appended path=w357:path)
            n275 = property class="VI"(reference=w352, error in=w351, "Front Panel Window:Open"=TRUE) -> (reference out=w349:refnum<vi>, error out=w350:errorcluster)
            n276 = Build Path(base path=w357, name or relative path=w348) -> (appended path=w355:path)
            n277 = Close Reference(reference=w349, error in (no error)=w350) -> (error out=w347:errorcluster)
            n278 = Unbundle By Name(w347) -> ("status"=w356:bool)
            n279 = case shown="True" w356 {
              tunnel: w355 -> [_ w359]
              tunnel: w347 -> [_ _]
              frame False {
              }
              frame True {
                n280 = stacked-sequence {
                  seq-local: [w365 _] -> [_ w372]
                  tunnel: w359 -> [_ w373]
                  frame #0 {
                    n281 = call "Setup_Filepath.vi"("Setup File Type"=Setup_Filetype."Calibration Setups", "Filename in"="Current_Setup.xls") -> ("Filename Out"=w360:path)  [unwired: 1 out]
                    n282 = call "Read_File_Simple.vi"("Filename"=w360) -> ("string"=w369:string)  [unwired: 2 in, 7 out]
                    n283 = Format Into String(format string="Calibration Setup File   %s", w360) -> (resulting string=w363:string)  [unwired: 2 in, 1 out]
                    n284 = call "Get_string_subset.vi"("String Name"=w363, "String to split"=w369, "File Label"="Raw data header") -> ("Output string"=w367:string)  [unwired: 1 in, 1 out]
                    n285 = call "Get_Characters_from_string.vi"("Input string"=w367, "Variable name"="Calib filename") -> ("Value"=w366:string)  [unwired: 1 in, 1 out]
                    n286 = call "String_to_Pathname.vi"("Input String"=w366) -> ("path"=w365:path)
                  }
                  frame #1 {
                    n287 = call "Does_file_exist_(simple).vi"("Pathname"=w372) -> ("exists?"=w371:bool)
                    n288 = case shown="True" w371 {
                      tunnel: w373 -> [w374 w389]
                      tunnel: w372 -> [_ w383]
                      frame False {
                        n289 = call "Open_Close_Front_Panel.ph.vi"("Front Panel Window:Open"=TRUE, "VI path"=w374) -> ()  [unwired: 2 out]
                      }
                      frame True {
                        w381 = TRUE ("Front Panel Window:Open")
                        n290 = Open VI Reference(type specifier VI Refnum (for type only)=refnum<vi> refnum, vi path=w389) -> (vi reference=w387:refnum<vi>, error out=w382:errorcluster)  [unwired: 1 in, 3 out]
                        n291 = property class="VI Interface Type 8"(reference=w387, error in=w382, "Front Panel Window:Open"=w381, "Front Panel Window:Auto Center (Deprecated)"=w381) -> (reference out=w386:refnum<vi>, error out=w385:errorcluster)
                        n292 = call-by-ref "?"(reference=w386, error in=w385, "Mode"=Calib_mode."Setup Front Panel", "Calib file"=w383) -> (reference out=w379:refnum<vi>, error out=w378:errorcluster)  [unwired: 15 in, 3 out]
                        n293 = property class="VI Interface Type 8"(reference=w379, error in=w378, "Front Panel Window:Auto Center (Deprecated)"=FALSE ("Front Panel Window:Auto Center")) -> (reference out=w377:refnum<vi>, error out=w376:errorcluster)
                        n294 = Close Reference(reference=w377, error in (no error)=w376) -> ()  [unwired: 1 out]
                      }
                    }
                  }
                }
              }
            }
            n295 = event-data() -> ()  [unwired: 1 in, 5 out]
          }
          event "stop": Mouse Down? {
            n296 = event-data() -> ()  [unwired: 5 out]
            n297 = flat-sequence {
              frame #0 {
                n298 = global write "Dynamic_call_global.ph.vi" "EnFlo Hub running?"(FALSE ("EnFlo Hub running?")) -> ()
              }
              frame #1 {
                n299 = Stop(stop? (T)=TRUE) -> ()
              }
            }
            n300 = event-data() -> ()  [unwired: 1 in, 4 out]
          }
          event "Rig_Control": Value Change {
            n301 = event-data() -> ("OldVal"=w393:cluster{"Ch Name":string, "Boolean":bool}[], "NewVal"=w392:cluster{"Ch Name":string, "Boolean":bool}[])  [unwired: 5 out]
            n302 = for {
              tunnel: w393 -> [w399] mode=indexing
              tunnel: w392 -> [w398] mode=indexing
              n303 = Unbundle By Name(w399) -> ("Ch Name"=w396:string, "Boolean"=w397:bool)
              n304 = Unbundle By Name(w398) -> ("Boolean"=w395:bool)  [unwired: 1 out]
              n305 = Not Equal?(x=w397, y=w395) -> (x != y?=w394:bool)
              n306 = case shown="True" w394 {
                tunnel: w396 -> [_ w401]
                tunnel: w395 -> [_ w408]
                frame False {
                }
                frame True {
                  n307 = Select(t="TRUE", s=w408, f="FALSE") -> (s? t:f=w400:string)
                  n308 = Select(t=1.0, s=w408, f=0.0) -> (s? t:f=w407:dbl)
                  n309 = Format Into String(format string="Are you sure you want to make %s %s?", w401, w400) -> (resulting string=w410:string)  [unwired: 2 in, 1 out]
                  n310 = Format Into String(format string="Make  %s  %s", w401, w400) -> (resulting string=w402:string)  [unwired: 2 in, 1 out]
                  n311 = Two Button Dialog(message=w410, 1:w402, 2:"Cancel" ("T button name (\"OK\")")) -> (T button?=w404:bool)
                  n312 = case shown="False" w404 {
                    tunnel: w401 -> [w415 _]
                    tunnel: w407 -> [w414 _]
                    frame False {
                      n313 = Build Array(w414) -> (w417:dbl[])
                      n314 = Build Array(w415) -> (w416:string[])
                      n315 = call "ASYNC_Adam_client.vi"("Values"=w417, "Channel Names"=w416) -> ()  [unwired: 2 out]
                    }
                    frame True {
                    }
                  }
                }
              }
            }
          }
        }
      }
    }
    "Numeric" <- w8
  }
  n316 = while {
    shift-left: _ -> [w422]
    shift-right: [w423] -> _
    shift-left: "Initialise" -> [w421]
    shift-right: [w424] -> _
    tunnel: "ADAM_Chs_to_Enable.txt" ("name or relative path") -> [w419]
    tunnel: "ADAM_Chs_to_View.txt" ("name or relative path") -> [w418]
    i -> [w420]
    stop <- TRUE continue-if-true
    n317 = case shown="\"Initialise\"" w421 {
      tunnel: ["End" "Initialise" "Wait for call remote sub vi occurrence" "Check type of VI to launch" w494 "Wait until remote sub vi is opened" "Update opened vis array" "Update opened vis array" "Update opened vis array" "Wait until remote sub vi is opened" "Wait for call remote sub vi occurrence"] -> w424
      tunnel: [w426 w439 w444 errorcluster {"status"=FALSE, "code"=0, "source"=""} ("error out") w490 w505 w535 w552 w567 w607 w627] -> w423
      tunnel: w422 -> [w426 w439 w444 _ w490 w505 _ _ _ w607 w627]
      tunnel: w421 -> [w428 _ _ _ _ _ _ _ _ _ _]
      tunnel: w420 -> [_ _ _ _ _ _ _ _ _ _ _]
      tunnel: w419 -> [_ _ w441 _ _ _ _ _ _ _ _]
      tunnel: w418 -> [_ _ w440 _ _ _ _ _ _ _ _]
      frame "No match", Default {
        n318 = Current VI's Path() -> (path=w429:path)
        n319 = Format Into String(format string="The Case\"%s\" was not Matched\nin VI named\n'%s\"" ("Format String"), w428, w429) -> (resulting string=w432:string)  [unwired: 2 in, 1 out]
        n320 = One Button Dialog(message=w432, button name ("OK")="STOP") -> (true=w430:bool)
        n321 = Stop(stop? (T)=w430) -> ()
      }
      frame "Never run" {
        # "These globals are here to make sure they stay in momory\nafter \"Preference Panel\" has finished running"
        n322 = call "Email_With_Log.vi"() -> ()  [unwired: 4 in, 3 out]
        n323 = call "Remember_value.vi"() -> ()  [unwired: 3 in, 1 out]
        n324 = call "Output_Trav_Pos.vi"() -> ()  [unwired: 5 in, 1 out]
        n325 = call "Read_Write_Local_table.vi"() -> ()  [unwired: 3 in, 3 out]
        n326 = call "Overhead_Factor.vi"() -> ()  [unwired: 4 in, 1 out]
        n327 = global read "Trav_pos_global.vi" "Dummy Measurement?"() -> (→"Dummy Measurement":bool)
        n328 = global read "PWAtasksGLOBAL.vi" "Analogue Dev Name"() -> (→"Analogue Dev Name":string)
        n329 = global read "Constants_global.vi" "All_Users"() -> (→"All Users":path)
        n330 = global read "Preference_global.vi" "Rig Setup"() -> (→"Rig Name":string)
      }
      frame "Initialise" {
        n331 = stacked-sequence {
          tunnel: w441 -> [_ _ _ _ w482]
          tunnel: w440 -> [_ _ _ _ w478]
          frame #0 {
            n332 = Generate Occurrence() -> (w465:refnum<k4>)
            n333 = global write "Dynamic_call_global.ph.vi" "Call Remote Subvi"(w465) -> ()
            n334 = Generate Occurrence() -> (w464:refnum<k4>)
            n335 = global write "Dynamic_call_global.ph.vi" "Remote Subvi Opened"(w464) -> ()
            n336 = Initialize Array("", 0) -> (w462:string[])
            n337 = global write "Dynamic_call_global.ph.vi" "Opened VIs"(w462) -> ()
            n338 = global write "Email_transfer_global.vi" "Busy?"(FALSE ("Busy?")) -> ()
            n339 = Current VI's Path() -> (path=w454:path)
            n340 = Strip Path(path=w454) -> (stripped path=w452:path)  [unwired: 1 out]
            n341 = Build Path(base path=w452, name or relative path="Utilities") -> (appended path=w450:path)
            n342 = Build Path(base path=w450, name or relative path="Preference_Panel.vi") -> (appended path=w449:path)
            n343 = Get Date/Time In Seconds() -> (seconds since 1Jan1904=w460:timestamp)
            n344 = To Double Precision Float(number=w460) -> (double precision float=w459:dbl)
            n345 = Open VI Reference(type specifier VI Refnum (for type only)=refnum<vi> refnum, vi path=w449) -> (vi reference=w455:refnum<vi>, error out=w456:errorcluster)  [unwired: 1 in, 3 out]
            n346 = global write "Meas_global.vi" "Start Time of experiment"(w459) -> ()
            n347 = global write "Meas_global.vi" "Post Process"(Post_Process."Post Process Raw Data File" ("Post Process")) -> ()
            n348 = call-by-ref "?"(reference=w455, error in=w456, "Mode"=Preference_Mode."Load Preferences from file") -> (reference out=w457:refnum<vi>, error out=w458:errorcluster)
            n349 = Close Reference(reference=w457, error in (no error)=w458) -> ()  [unwired: 1 out]
          }
          frame #1 {
            w466 = TRUE  # OK
            n350 = call "Get_users_email_addresses.vi"("OK"=w466) -> ()  [unwired: 5 out]
          }
          frame #2 {
            n351 = Current VI's Path() -> (path=w475:path)
            n352 = Open VI Reference(vi path=w475) -> (vi reference=w474:refnum<vi>, error out=w473:errorcluster)  [unwired: 1 in, 4 out]
            n353 = call "Last_modified_date.vi"("Update Now"=TRUE) -> ("RevisionString"=w467:string)  [unwired: 1 out]
            n354 = property class="VI"(reference=w474, error in=w473, "Front Panel Window:Open"=TRUE, "Front Panel Window:Is Frontmost"=FALSE) -> (reference out=w472:refnum<vi>, error out=w471:errorcluster)
            n355 = global write "Meas_global.vi" "ProgRevisionInfo"(w467) -> ()
            n356 = Close Reference(reference=w472, error in (no error)=w471) -> ()  [unwired: 1 out]
          }
          frame #3 {
            n357 = global write "Dynamic_call_global.ph.vi" "EnFlo Hub running?"(TRUE ("EnFlo Hub running?")) -> ()
          }
          frame #4 {
            n358 = global read "Constants_global.vi" "All_Users"() -> (w479:path)
            n359 = Build Path(base path=w479, name or relative path=w478) -> (appended path=w481:path)
            n360 = Build Path(base path=w479, name or relative path=w482) -> (appended path=w484:path)
            n361 = call "Read_File_Simple.vi"("Filename"=w481) -> ("string"=w480:string)  [unwired: 2 in, 7 out]
            n362 = call "Read_File_Simple.vi"("Filename"=w484) -> ("string"=w485:string)  [unwired: 2 in, 7 out]
            n363 = call "Get_array_values_fr_String.vi"("String Value"=w480) -> ("String array"=→"List of ADAM channels to view":string[])  [unwired: 1 out]
            n364 = call "Get_array_values_fr_String.vi"("String Value"=w485) -> ("String array"=→"List of ADAM control channels":string[])  [unwired: 1 out]
          }
        }
        "Iterations" <- 0 ("Iterations")
      }
      frame "Wait for call remote sub vi occurrence" {
        n365 = global read "Dynamic_call_global.ph.vi" "Call Remote Subvi"() -> (w488:refnum<k4>)
        n366 = Wait on Occurrence(2:w488) -> ()  [unwired: 3 out]
      }
      frame "Check type of VI to launch" {
        n367 = global read "Dynamic_call_global.ph.vi" "VI name to launch"() -> (w492:string)
        n368 = Match Pattern(string=w492, regular expression=";") -> (before substring=w489:string, after substring=w491:string)  [unwired: 3 out]
        n369 = case shown="\"Open LDA PWA & An\"" w489 {
          tunnel: ["Open vi" "Open application reference" "Open Analogue input server" w502] -> w494
          tunnel: [w497 w499 w501 w503] -> w493
          tunnel: w492 -> [w497 _ _ _]
          tunnel: w491 -> [_ w499 w501 w503]
          tunnel: w489 -> [_ _ _ w502]
          frame "Other", Default {
          }
          frame "Open Application Reference" {
          }
          frame "Open Analogue Input VI" {
          }
          frame "Open LDA PWA & An" {
          }
        }
        "VI Name" <- w493
      }
      frame "Open application reference" {
        n370 = local read "VI Name"() -> (w506:string)
        n371 = Match Pattern(string=w506, regular expression=";") -> (before substring=w514:string, after substring=w515:string)  [unwired: 3 out]
        n372 = Decimal String To Number(string=w515) -> (number=w516:i32)  [unwired: 3 out]
        n373 = To Unsigned Long Integer(number=w516) -> (unsigned 32bit integer=w513:u32)
        n374 = call "App_Ref_Global.vi"("Mode"=App_Global."Read Global") -> ("Output Array"=w512:T48[])  [unwired: 1 in, 1 out]
        n375 = Open Application Reference(10:w513, 11:w514) -> (0:w507:errorcluster, 3:w511:refnum<vi>)  [unwired: 1 in, 1 out]
        n376 = for {
          tunnel: w512 -> [w518] mode=indexing
          tunnel: w506 -> [w522]
          tunnel: w511 -> [w520]
          tunnel: [w519] -> w510 mode=indexing
          n377 = Unbundle By Name(w518) -> ("Server IP & Port No"=w523:string)
          n378 = Equal?(x=w523, y=w522) -> (x = y?=w521:bool)
          n379 = case shown="False" w521 {
            tunnel: w520 -> [_ w527]
            tunnel: [w524 w526] -> w519
            tunnel: w518 -> [w524 w525]
            frame False {
            }
            frame True {
              n380 = Bundle By Name(cluster=w525, "Application reference"=w527) -> (w526:T48)
            }
          }
        }
        n381 = global write "Dynamic_call_global.ph.vi" "Error Cluster"(w507) -> ()
        n382 = call "App_Ref_Global.vi"("Input Array"=w510, "Mode"=App_Global."Write to Global") -> ()  [unwired: 2 out]
      }
      frame "Open Analogue input server" {
        n383 = local read "VI Name"() -> (w532:string)
        n384 = call "Get_link_info.vi"("VI Name"=w532) -> ("Path name"=w529:path, "Application reference"=w530:refnum<vi>, "Local Call?"=w531:bool)  [unwired: 1 out]
        n385 = global read "Dynamic_call_global.ph.vi" "Analogue Input"() -> (w534:refnum<vi>)
        n386 = case shown="True" w531 {
          tunnel: w534 -> [w540 w544]
          tunnel: [w536 w543] -> w533
          tunnel: [w539 w542] -> w535
          tunnel: w532 -> [w538 _]
          tunnel: w530 -> [w537 _]
          tunnel: w529 -> [_ w541]
          frame False {
            n387 = Open VI Reference(type specifier VI Refnum (for type only)=w540, application reference (local)=w537, vi path=w538) -> (vi reference=w536:refnum<vi>, error out=w539:errorcluster)  [unwired: 1 in, 2 out]
          }
          frame True {
            n388 = Open VI Reference(type specifier VI Refnum (for type only)=w544, vi path=w541) -> (vi reference=w543:refnum<vi>, error out=w542:errorcluster)  [unwired: 1 in, 3 out]
          }
        }
        n389 = global write "Dynamic_call_global.ph.vi" "Analogue Input"(w533) -> ()
      }
      frame "Open LDA PWA & An" {
        n390 = local read "VI Name"() -> (w549:string)
        n391 = call "Get_link_info.vi"("VI Name"=w549) -> ("Path name"=w546:path, "Application reference"=w547:refnum<vi>, "Local Call?"=w548:bool)  [unwired: 1 out]
        n392 = global read "Dynamic_call_global.ph.vi" "Take LDA PWA & An"() -> (w551:refnum<vi>)
        n393 = case shown="True" w548 {
          tunnel: w551 -> [w557 w561]
          tunnel: [w553 w560] -> w550
          tunnel: [w556 w559] -> w552
          tunnel: w549 -> [w555 _]
          tunnel: w547 -> [w554 _]
          tunnel: w546 -> [_ w558]
          frame False {
            n394 = Open VI Reference(type specifier VI Refnum (for type only)=w557, application reference (local)=w554, vi path=w555) -> (vi reference=w553:refnum<vi>, error out=w556:errorcluster)  [unwired: 1 in, 2 out]
          }
          frame True {
            n395 = Open VI Reference(type specifier VI Refnum (for type only)=w561, vi path=w558) -> (vi reference=w560:refnum<vi>, error out=w559:errorcluster)  [unwired: 1 in, 3 out]
          }
        }
        n396 = global write "Dynamic_call_global.ph.vi" "Take LDA PWA & An"(w550) -> ()
      }
      frame "Open vi" {
        n397 = local read "VI Name"() -> (w566:string)
        n398 = call "Get_link_info.vi"("VI Name"=w566) -> ("Path name"=w565:path, "Application reference"=w564:refnum<vi>, "Local Call?"=w563:bool)  [unwired: 1 out]
        n399 = case shown="\"No Match\", Default" w566 {
          tunnel: [w568 w577 w589] -> w567
          tunnel: w566 -> [w573 w576 w593]
          tunnel: w565 -> [_ _ w590]
          tunnel: w564 -> [_ w575 w592]
          tunnel: w563 -> [_ w574 w591]
          frame "No Match", Default {
            n400 = Format Into String(format string="VI named \"%s\" Not matched" ("Format String"), w573) -> (resulting string=w570:string)  [unwired: 2 in, 1 out]
            n401 = Bundle By Name(cluster=errorcluster {"status"=FALSE, "code"=0, "source"=""} ("error out"), "source"=w570, "status"=TRUE ("Bundle Element")) -> (w568:errorcluster)
          }
          frame "Program_Active_server.vi" {
            n402 = global read "Dynamic_call_global.ph.vi" "Program Active server"() -> (w579:refnum<vi>)
            n403 = case shown="True" w574 {
              tunnel: w579 -> [w584 w588]
              tunnel: [w583 w587] -> w578
              tunnel: [w582 w586] -> w577
              tunnel: w576 -> [w581 w585]
              tunnel: w575 -> [w580 _]
              frame False {
                n404 = Open VI Reference(type specifier VI Refnum (for type only)=w584, application reference (local)=w580, vi path=w581) -> (vi reference=w583:refnum<vi>, error out=w582:errorcluster)  [unwired: 1 in, 2 out]
              }
              frame True {
                n405 = Open VI Reference(type specifier VI Refnum (for type only)=w588, vi path=w585) -> (vi reference=w587:refnum<vi>, error out=w586:errorcluster)  [unwired: 1 in, 3 out]
              }
            }
            n406 = global write "Dynamic_call_global.ph.vi" "Program Active server"(w578) -> ()
          }
          frame "GPIB_Server.vi" {
            n407 = global read "Dynamic_call_global.ph.vi" "GPIB_Server.vi"() -> (w595:refnum<vi>)
            n408 = case shown="False" w591 {
              tunnel: w595 -> [w600 w604]
              tunnel: [w599 w603] -> w594
              tunnel: [w598 w602] -> w589
              tunnel: w593 -> [w596 _]
              tunnel: w592 -> [w597 _]
              tunnel: w590 -> [_ w601]
              frame False {
                n409 = Open VI Reference(type specifier VI Refnum (for type only)=w600, application reference (local)=w597, vi path=w596) -> (vi reference=w599:refnum<vi>, error out=w598:errorcluster)  [unwired: 1 in, 2 out]
              }
              frame True {
                n410 = Open VI Reference(type specifier VI Refnum (for type only)=w604, vi path=w601) -> (vi reference=w603:refnum<vi>, error out=w602:errorcluster)  [unwired: 1 in, 3 out]
              }
            }
            n411 = global write "Dynamic_call_global.ph.vi" "GPIB_Server.vi"(w594) -> ()
          }
        }
      }
      frame "Update opened vis array" {
        w609 = TRUE  # Dialog Box
        n412 = local read "VI Name"() -> (w608:string)
        n413 = Unbundle By Name(w607) -> ("status"=w612:bool, "source"=w610:string)
        n414 = case shown="True" w612 {
          tunnel: w607 -> [w614 w623]
          tunnel: [w614 w622] -> w611
          tunnel: w608 -> [w615 w618]
          tunnel: w610 -> [_ w621]
          frame False {
            n415 = To Upper Case(1:w615) -> (0:w613:string)
            n416 = global read "Dynamic_call_global.ph.vi" "Opened VIs"() -> (w616:string[])
            n417 = Build Array (concatenate)(w616, w613) -> (w617:string[])
            n418 = global write "Dynamic_call_global.ph.vi" "Opened VIs"(w617) -> ()
          }
          frame True {
            n419 = Concatenate Strings(w618, " " ("Substring"), w621) -> (w619:string)
            n420 = Bundle By Name(cluster=w623, "source"=w619) -> (w622:errorcluster)
          }
        }
        n421 = call "EnFlo_Error_Handler.vi"("error in (no error)"=w611, "Error Type"="Dynamic Call", "Dialog Box (T)"=w609) -> ()  [unwired: 3 out]
      }
      frame "Wait until remote sub vi is opened" {
        n422 = global read "Dynamic_call_global.ph.vi" "Remote Subvi Opened"() -> (w628:refnum<k4>)
        n423 = local read "Iterations"() -> (w626:i32)
        n424 = Increment(x=w626) -> (x+1=w625:i32)
        n425 = local write "Iterations"(w625) -> ()
        n426 = Set Occurrence(w628) -> ()
      }
    }
  }
  n427 = while {
    i -> [w629]
    stop <- FALSE stop-if-true
    n428 = stacked-sequence {
      tunnel: w629 -> [_ w676]
      frame #0 {
        n429 = global read "Dynamic_call_global.ph.vi" "EnFlo Hub running?"() -> (w633:bool)
        n430 = Equal?(x="Tab Control", y=T1."Adam Table" ("Tab Control")) -> (x = y?=w634:bool)
        n431 = And(x=w634, y=w633) -> (x .and. y?=w632:bool)
        n432 = case shown="True" w632 {
          frame True {
            n433 = local read "List of ADAM channels to view"() -> (w643:string[])
            n434 = local read "List of ADAM control channels"() -> (w646:string[])
            n435 = Build Array (concatenate)(w646, w643) -> (w645:string[])
            n436 = call "Get_Current_Scan_client.vi"("ADAM Ch Names"=w645) -> ("Ch Description Array"=w640:T50[], "Numerical Values"=w644:dbl[])  [unwired: 2 out]
            n437 = Array Size(array=w646) -> (size(s)=w641:i32)
            n438 = Array Subset(array=w640, index=w641) -> (w639:T50[])  [unwired: 1 in]
            n439 = Array Subset(array=w644, index=w641) -> (w638:dbl[])  [unwired: 1 in]
            n440 = for {
              tunnel: w639 -> [w653] mode=indexing
              tunnel: [w652] -> w637 mode=indexing
              tunnel: cluster{"Ch Name":string, "Numeric":dbl} {"Ch Name"="", "Numeric"=0.0} ("Cluster") -> [w651]
              tunnel: w638 -> [w649] mode=indexing
              n441 = Unbundle By Name(w653) -> ("Ch Name"=w650:string)
              n442 = Bundle By Name(cluster=w651, "Ch Name"=w650, "Numeric"=w649) -> (w652:cluster{"Ch Name":string, "Numeric":dbl})
            }
            "Current Values" <- w637
            n443 = for {
              N: w641 -> [_]
              tunnel: cluster{"Ch Name":string, "Boolean":bool} {"Ch Name"="", "Boolean"=FALSE} ("Cluster") -> [w660]
              tunnel: w640 -> [w659] mode=indexing
              tunnel: w644 -> [w657] mode=indexing
              tunnel: [w654] -> w647 mode=indexing
              n444 = Unbundle By Name(w659) -> ("Ch Name"=w658:string)
              n445 = Greater?(x=w657, y=0.5) -> (0:w655:bool)
              n446 = Bundle By Name(cluster=w660, "Ch Name"=w658, "Boolean"=w655) -> (w654:cluster{"Ch Name":string, "Boolean":bool})
            }
            n447 = local write "Rig_Control"(w647) -> ()
          }
          frame False {
          }
        }
      }
      frame #1 {
        w674 = 300 ("y")
        n448 = Quotient & Remainder(x=w676, y=3600) -> (x-y*floor(x/y)=w677:i32)  [unwired: 1 out]
        n449 = Quotient & Remainder(x=w676, y=900) -> (x-y*floor(x/y)=w673:i32)  [unwired: 1 out]
        n450 = Equal?(x=w677, y=w674) -> (x = y?=w671:bool)
        n451 = Equal?(x=w674, y=w673) -> (x = y?=w672:bool)
        n452 = Or(x=w671, y=w672) -> (x .or. y?=w664:bool)
        n453 = Select(t=3 ("Months of History to backup"), s=w671, f=0) -> (s? t:f=w668:i32)
        n454 = global read "Preference_global.vi" "Server Comms"() -> (w666:T49)
        n455 = Equal?(x=w666, y=Server_Comms."Server Link Healthy" ("Server Comms")) -> (x = y?=w665:bool)
        n456 = And(x=w664, y=w665) -> (x .and. y?=w662:bool)
        n457 = Or(x="Sync to server now", y=w662) -> (x .or. y?=w661:bool)
        n458 = case shown="True" w661 {
          tunnel: w668 -> [_ w679]
          frame False {
          }
          frame True {
            n459 = stacked-sequence {
              tunnel: w679 -> [w682 _]
              frame #0 {
                w680 = TRUE  # Check Updates on Server?
                w681 = TRUE  # Get all Server Files
                n460 = call "Backup_Client.vi"("Check Updates on Server?"=w680, "Get all Server Files"=w681, "Months of History to backup"=w682) -> ()  [unwired: 1 out]
              }
              frame #1 {
                n461 = local write "Sync to server now"(FALSE ("Sync to server now")) -> ()
              }
            }
          }
        }
      }
    }
    n462 = Wait (ms)(milliseconds to wait=u32 1000) -> ()  [unwired: 1 out]
  }
